vi "端铆试验判定.vi"(7 "Result":refnum<vi>, 9 "判定参数":T1, 10 "XY曲线 2":cluster{"X":dbl[], "Y":dbl[]}[](array[cluster]), 11 "XY曲线":cluster{"X":dbl[], "Y":dbl[]}[](array[cluster])) -> (2 "判定项长度":i32, 3 "OK？":bool)   [LabVIEW 2020]
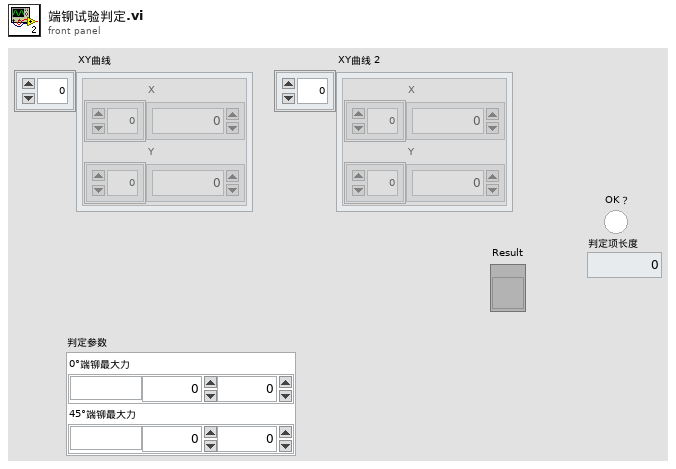
[diagram p1: front panel]
types:
  T1 = cluster{"0°端铆最大力":cluster{"单位":string, "下限":dbl, "上限":dbl}, "45°端铆最大力":cluster{"单位":string, "下限":dbl, "上限":dbl}}
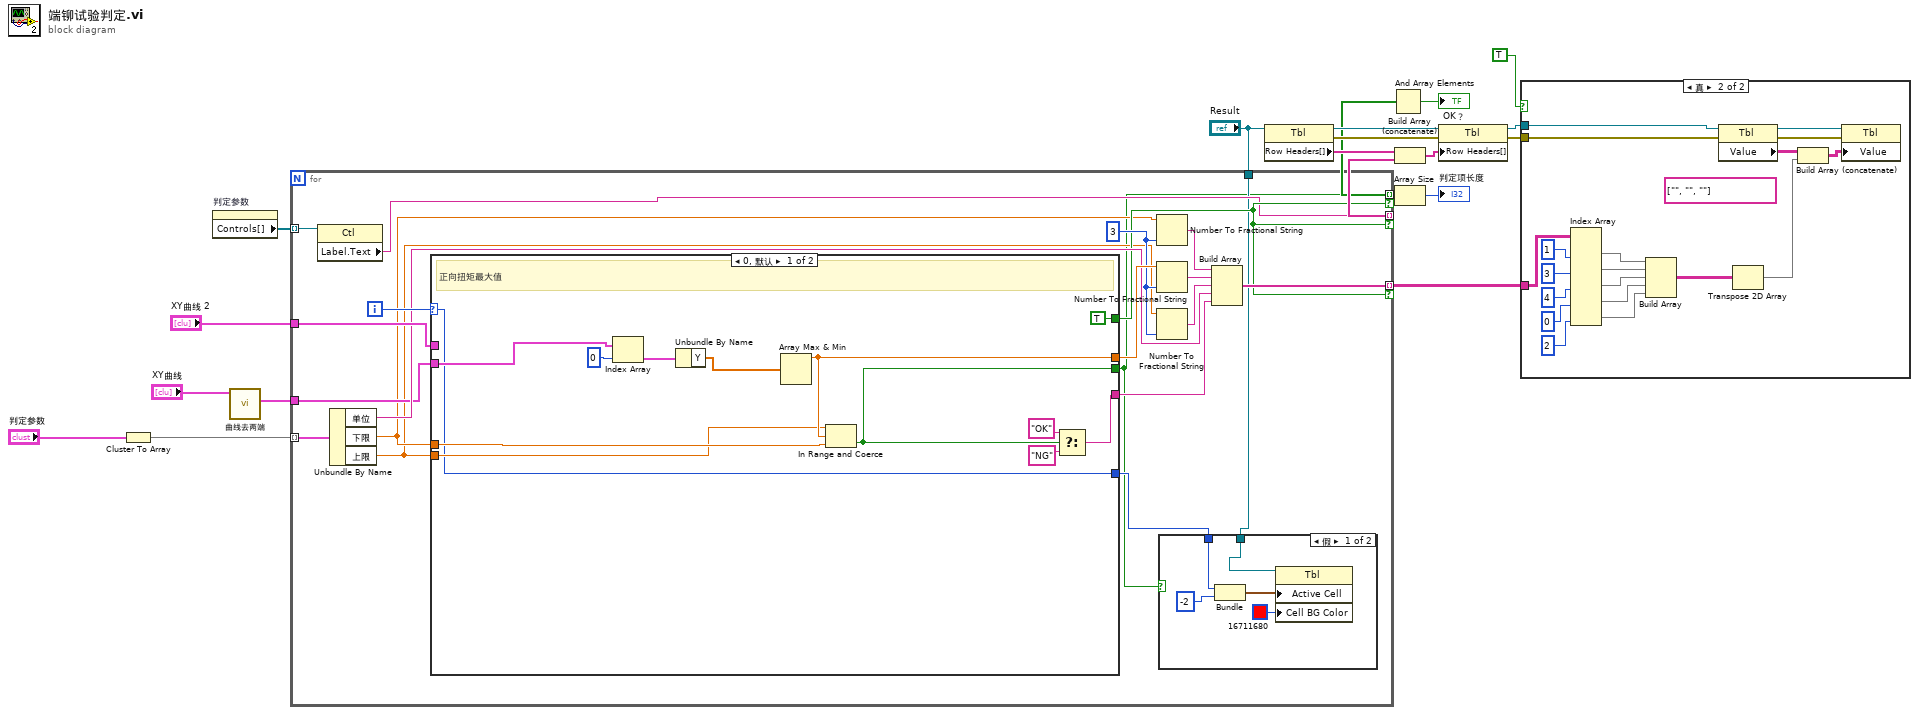
[diagram p0: block diagram]
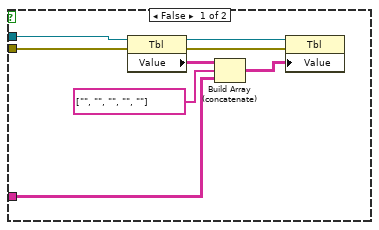
[diagram p2: hidden frame]
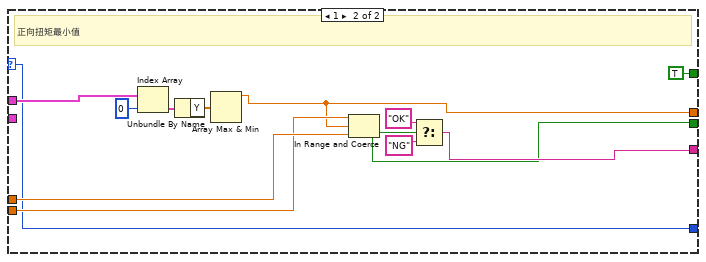
[diagram p4: hidden frame]
diagram:
  n1 = Cluster To Array(cluster="判定参数") -> (array=w19:cluster{"单位":string, "下限":dbl, "上限":dbl}[])
  n2 = property on="判定参数" class="Clust (严格)"() -> ("Controls[]"=w9:refnum<vi>[])  [unwired: 2 in, 2 out]
  n3 = call "曲线去两端.vi"("曲线In"="XY曲线") -> ("启动曲线"=w5:cluster{"X":dbl[], "Y":dbl[]}[])  [unwired: 9 in, 1 out]
  n4 = for {
    tunnel: w19 -> [w39] mode=indexing
    tunnel: w9 -> [w37] mode=indexing
    tunnel: "XY曲线 2" -> [w35]
    tunnel: [w20] -> w7 mode=indexing if=w27
    tunnel: [w28] -> w10 mode=indexing if=w27
    tunnel: [w23] -> w12 mode=indexing if=w27
    tunnel: w5 -> [w26]
    tunnel: "Result" -> [w22]
    i -> [w38]
    w34 = i16 3 ("精度(6)")
    n5 = property class="Ctl"(reference=w37) -> ("Label.Text"=w23:string)  [unwired: 1 in, 2 out]
    n6 = Unbundle By Name(w39) -> ("单位"=w29:string, "下限"=w25:dbl, "上限"=w24:dbl)
    n7 = case shown="0, 默认" w38 {
      selector: w38 -> [w45 w58]
      tunnel: [w55 w59] -> w36
      tunnel: w35 -> [_ w70]
      tunnel: [w52 w66] -> w30
      tunnel: [w51 w65] -> w20
      tunnel: w25 -> [w50 w64]
      tunnel: w24 -> [w49 w63]
      tunnel: [TRUE TRUE] -> w27
      tunnel: w26 -> [w46 _]
      tunnel: [w45 w58] -> w21
      frame 0, Default {
        # "正向扭矩最大值"
        n8 = Index Array(array=w46, index=0 ("索引")) -> (element=w56:cluster{"X":dbl[], "Y":dbl[]})
        n9 = Unbundle By Name(w56) -> ("Y"=w47:dbl[])
        n10 = Array Max & Min(array=w47) -> (max value=w55:dbl)  [unwired: 3 out]
        n11 = In Range and Coerce(upper limit=w49, x=w55, lower limit=w50) -> (In Range?=w51:bool)  [unwired: 1 out]
        n12 = Select(t="OK", s=w51, f="NG") -> (s? t:f=w52:string)
      }
      frame 1 {
        # "正向扭矩最小值"
        n13 = Index Array(array=w70, index=0 ("索引")) -> (element=w69:cluster{"X":dbl[], "Y":dbl[]})
        n14 = Unbundle By Name(w69) -> ("Y"=w61:dbl[])
        n15 = Array Max & Min(array=w61) -> (max value=w59:dbl)  [unwired: 3 out]
        n16 = In Range and Coerce(upper limit=w63, x=w59, lower limit=w64) -> (In Range?=w65:bool)  [unwired: 1 out]
        n17 = Select(t="OK", s=w65, f="NG") -> (s? t:f=w66:string)
      }
    }
    n18 = Number To Fractional String(number=w25, precision (6)=w34) -> (F-format string=w33:string)  [unwired: 2 in]
    n19 = Number To Fractional String(number=w36, precision (6)=w34) -> (F-format string=w32:string)  [unwired: 2 in]
    n20 = Number To Fractional String(number=w24, precision (6)=w34) -> (F-format string=w31:string)  [unwired: 2 in]
    n21 = case shown="假" w20 {
      tunnel: w22 -> [w44 _]
      tunnel: w21 -> [w40 _]
      frame False {
        n22 = Bundle(w40, "索引"=-2) -> (w41:cluster{i32, "索引":i32})  [unwired: 1 in]
        n23 = property class="Tbl"(reference=w44, "Active Cell"=w41, "Cell BG Color"=u32 16711680 ("活动单元格:单元格背景色")) -> ()  [unwired: 1 in, 2 out]
      }
      frame True {
      }
    }
    n24 = Build Array(w33, w32, w31, w29, w30) -> (w28:string[])
  }
  n25 = property class="Tbl"(reference="Result") -> (reference out=w14:refnum<vi>, error out=w17:errorcluster, "Row Headers[]"=w11:string[])  [unwired: 1 in]
  n26 = And Array Elements(Boolean array=w7) -> (logical AND=→"OK？":bool)
  n27 = Build Array (concatenate)(w11, w12) -> (w13:string[])
  n28 = Array Size(array=w7) -> (size(s)=→"判定项长度":i32)
  n29 = property class="Tbl"(reference=w14, error in=w17, "Row Headers[]"=w13) -> (reference out=w15:refnum<vi>, error out=w16:errorcluster)
  n30 = case shown="真" TRUE {
    tunnel: w16 -> [w76 w95]
    tunnel: w15 -> [w73 w92]
    tunnel: w10 -> [w72 w91]
    frame False {
      n31 = property class="Tbl"(reference=w73, error in=w76) -> (reference out=w74:refnum<vi>, error out=w75:errorcluster, "Value"=w77:string[][])
      n32 = Build Array (concatenate)(w77, string[] ["", "", "", "", ""], w72) -> (w78:string[][])
      n33 = property class="Tbl"(reference=w74, error in=w75, "Value"=w78) -> ()  [unwired: 2 out]
    }
    frame True {
      (unwired) string[] ["", "", ""]
      n34 = Index Array(array=w91, index (col) #1=1 ("禁用的索引 (列)"), index (col) #2=3 ("索引 (列)"), index (col) #3=4 ("索引 (列)"), index (col) #4=0 ("索引 (列)"), index (col) #5=2 ("索引 (列)")) -> (element #1=w87:string[], element #2=w86:string[], element #3=w85:string[], element #4=w80:string[], element #5=w79:string[])  [unwired: 5 in]
      n35 = Build Array(w87, w86, w85, w80, w79) -> (w84:string[][])
      n36 = property class="Tbl"(reference=w92, error in=w95) -> (reference out=w93:refnum<vi>, error out=w94:errorcluster, "Value"=w96:string[][])
      n37 = Transpose 2D Array(2D array=w84) -> (transposed array=w83:string[][])
      n38 = Build Array (concatenate)(w96, w83) -> (w97:string[][])
      n39 = property class="Tbl"(reference=w93, error in=w94, "Value"=w97) -> ()  [unwired: 2 out]
    }
  }
